vi "Extra Awesome Autonomous.vi"() -> ()   [LabVIEW 2013]
panel:
  in  "Move 2":i32=500
  in  "Move":i32=500
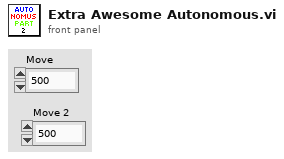
[diagram p1: front panel]
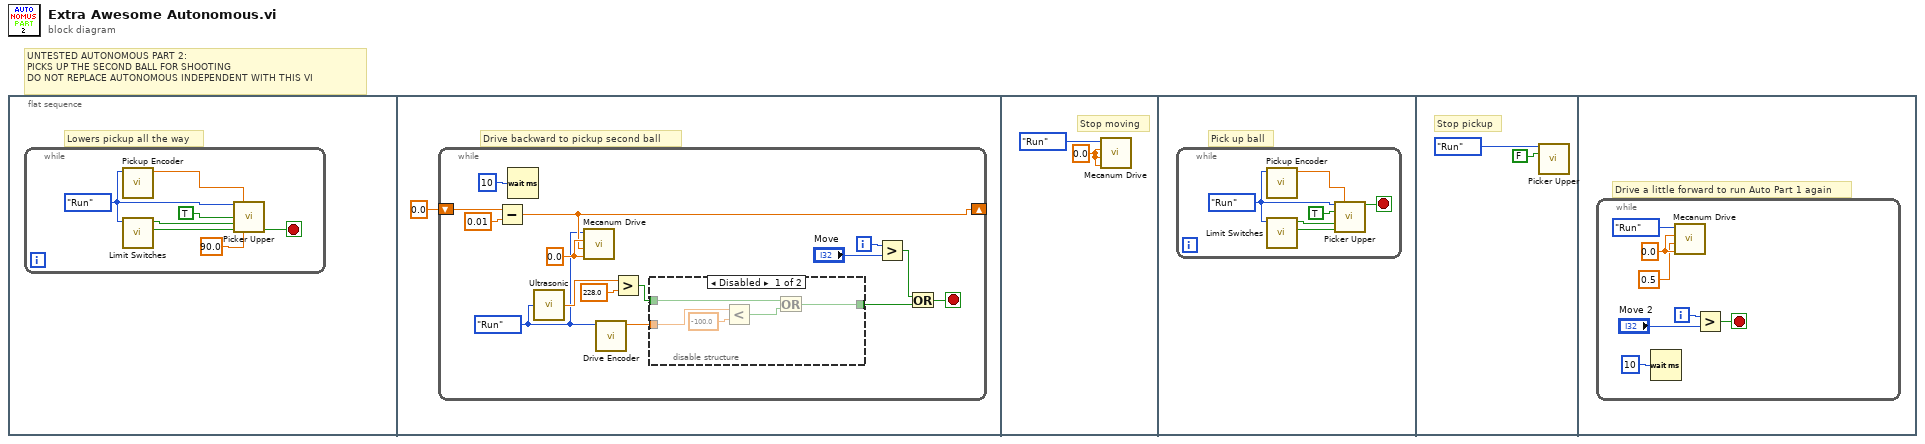
[diagram p0: block diagram]
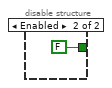
[diagram p2: hidden frame]
diagram:
  # "UNTESTED AUTONOMOUS PART 2:\nPICKS UP THE SECOND BALL FOR SHOOTING\nDO NOT REPLACE AUTONOMOUS INDEPENDENT WITH THIS VI"
  n1 = flat-sequence {
    frame #0 {
      # "Lowers pickup all the way"
      n2 = while {
        stop <- w7 stop-if-true
        w5 = enum16{"Open", "Run", "End"}."Run" ("State Control")
        n3 = call "Pickup Encoder.vi"("State Control"=w5) -> ("Encoder Degrees"=w4:dbl)  [unwired: 3 in, 3 out]
        n4 = call "Limit Switches.vi"("State Control"=w5) -> ("Picker Upper Bottom"=w6:bool, "Picker Upper Top"=w2:bool)  [unwired: 7 in, 2 out]
        n5 = call "Picker Upper.vi"("State Control"=w5, "Encoder"=w4, "Down"=TRUE, "Top limit"=w2, "Bottom Limit"=w6, "Down break"=90.0 ("Down break 2")) -> ("Fully down?"=w7:bool)  [unwired: 8 in, 1 out]
      }
    }
    frame #1 {
      # "Drive backward to pickup second ball"
      n6 = while {
        shift-right: [w11] -> _
        shift-left: 0.0 ("Strafing") -> [w13]
        i -> [w23]
        stop <- w16 stop-if-true
        w20 = 0.0 ("Strafing")
        w10 = enum16{"Open", "Run", "End"}."Run" ("State Control")
        n7 = Subtract(x=w13, y=0.01) -> (x-y=w11:dbl)
        n8 = Wait (ms)(milliseconds to wait=u32 10) -> ()  [unwired: 1 out]
        n9 = call "Ultrasonic.vi"("State Control"=w10) -> ("Distance (in.)"=w19:dbl)
        n10 = call "Mecanum Drive.vi"("Turn"=w20, "Forward/Backward"=w11, "Strafe"=w20, "State Control"=w10) -> ()  [unwired: 4 in]
        n11 = call "Drive Encoder.vi"("State Control"=w10) -> ("Encoder Degrees"=w9:dbl)  [unwired: 3 in, 3 out]
        n12 = Greater?(x=w19, y=228.0) -> (0:w14:bool)
        n13 = disable-structure shown="Disabled" {
          disable-tunnel: [w24 FALSE] -> w15
          disable-tunnel: w14 -> [w25 _]
          disable-tunnel: w9 -> [w28 _]
          frame Disabled {
            n14 = Less?(x=w28, y=-100.0) -> (x < y?=w26:bool)
            n15 = Or(x=w25, y=w26) -> (x .or. y?=w24:bool)
          }
          frame Enabled {
          }
        }
        n16 = Greater?(x=w23, y="Move") -> (0:w17:bool)
        n17 = Or(x=w17, y=w15) -> (x .or. y?=w16:bool)
      }
    }
    frame #2 {
      w30 = 0.0 ("F/R")
      # "Stop moving"
      n18 = call "Mecanum Drive.vi"("Turn"=w30, "Forward/Backward"=w30, "Strafe"=w30, "State Control"=enum16{"Open", "Run", "End"}."Run") -> ()  [unwired: 4 in]
    }
    frame #3 {
      # "Pick up ball"
      n19 = while {
        stop <- w32 stop-if-true
        w36 = enum16{"Open", "Run", "End"}."Run" ("State Control")
        n20 = call "Pickup Encoder.vi"("State Control"=w36) -> ("Encoder Degrees"=w35:dbl)  [unwired: 3 in, 3 out]
        n21 = call "Limit Switches.vi"("State Control"=w36) -> ("Picker Upper Bottom"=w37:bool, "Picker Upper Top"=w34:bool)  [unwired: 7 in, 2 out]
        n22 = call "Picker Upper.vi"("State Control"=w36, "Encoder"=w35, "Up"=TRUE ("Down"), "Top limit"=w34, "Bottom Limit"=w37) -> ("Fully up?"=w32:bool)  [unwired: 9 in, 1 out]
      }
    }
    frame #4 {
      # "Stop pickup"
      n23 = call "Picker Upper.vi"("State Control"=enum16{"Open", "Run", "End"}."Run", "Up"=FALSE ("Down")) -> ()  [unwired: 12 in, 2 out]
    }
    frame #5 {
      # "Drive a little forward to run Auto Part 1 again"
      n24 = while {
        i -> [w46]
        stop <- w40 stop-if-true
        w43 = 0.0 ("Strafing")
        n25 = Wait (ms)(milliseconds to wait=u32 10) -> ()  [unwired: 1 out]
        n26 = call "Mecanum Drive.vi"("Turn"=w43, "Forward/Backward"=0.5 ("y"), "Strafe"=w43, "State Control"=enum16{"Open", "Run", "End"}."Run") -> ()  [unwired: 4 in]
        n27 = Greater?(x=w46, y="Move 2") -> (0:w40:bool)
      }
    }
  }
